vi "Abort Trigger.vi"(8 "error in":errorcluster, 11 "VISA resource name in":refnum<visa-resource-name>) -> (0 "error out":errorcluster, 3 "VISA resource name out":refnum<visa-resource-name>)   [LabVIEW 2021, in "Keysight U1282A.lvlib"]
doc: "El comando abortar (ABOR) coloca el instrumento U1282A en el estado de espera cuando se encuentra en el modo trigger hold. La pantalla del instrumento mostrará (-) hasta que el comando INIT sea utilizado."
uses:
  Keysight U1282A.lvlib
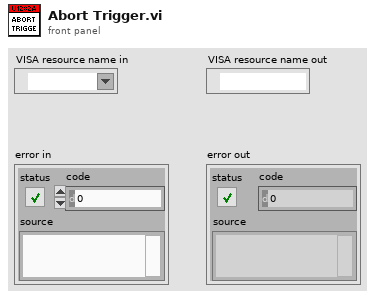
[diagram p1: front panel]
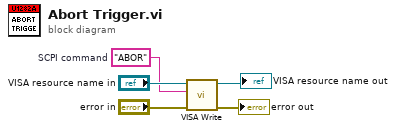
[diagram p0: block diagram]
diagram:
  w1 = "ABOR"  # SCPI command
  n1 = call "VISA Write.vi"("error in"="error in", "SCPI command"=w1, "VISA resource in"="VISA resource name in") -> ("error out"=→"error out":errorcluster, "VISA resource out"=→"VISA resource name out":refnum<visa-resource-name>)  [unwired: 6 in, 1 out]
